vi "Init.vi"(8 "error in":errorcluster, 9 "Values":refnum<class "Value.lvclass">[](array[class]), 10 "Keys":refnum<class "Key Name.lvclass">[](array[class]), 11 "VAR in":refnum<class "VAR.lvclass">) -> (0 "error out":errorcluster, 3 "VAR out":refnum<class "VAR.lvclass">)   [LabVIEW 2020, in "Electronic Datasheet.lvlib" / "VAR.lvclass"]
uses:
  VAR.lvclass
  Keyname/Key Name.lvclass
  Value/Value.lvclass
  Object Type/Object Type Base.lvclass
  Electronic Datasheet.lvlib
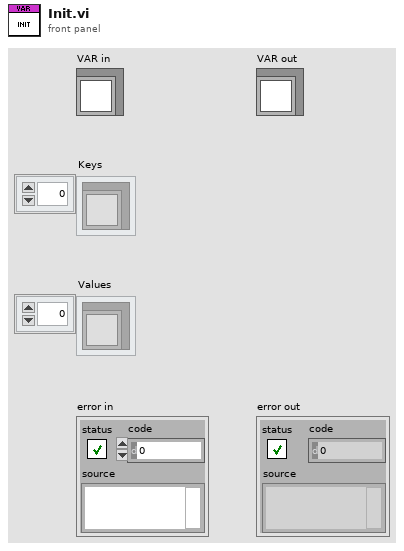
[diagram p1: front panel]
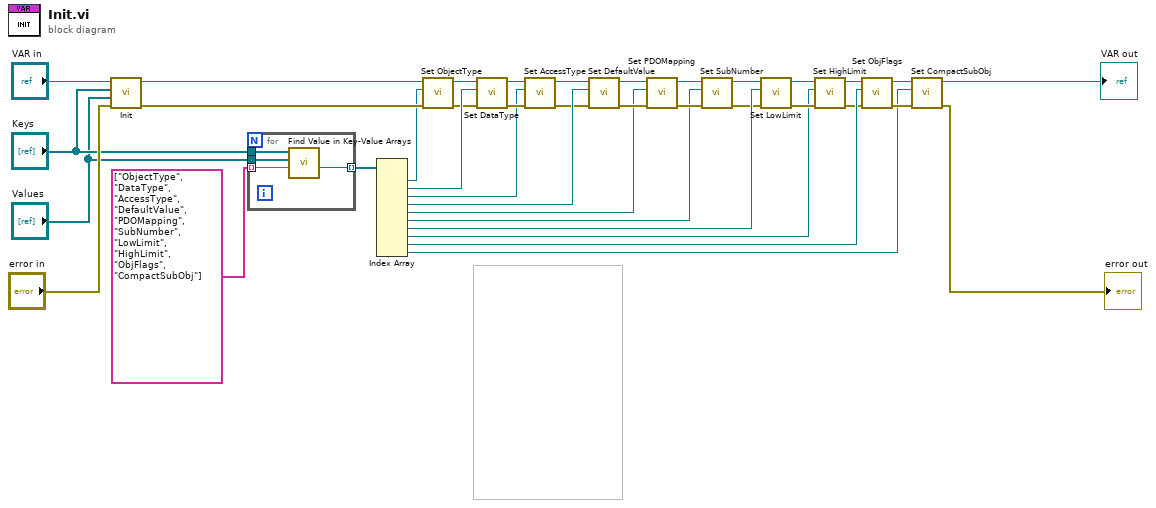
[diagram p0: block diagram]
diagram:
  n1 = call-parent "Init.vi"("error in"="error in", "Values"="Values", "Keys"="Keys", "Object Type in"="VAR in") -> ("error out"=w36:errorcluster, "Object Type out"=w3:refnum<class "VAR.lvclass">)  [unwired: 6 in]
  n2 = for {
    tunnel: "Keys" -> [w42]
    tunnel: "Values" -> [w41]
    tunnel: [w40] -> w32 mode=indexing
    tunnel: string[] ["ObjectType", "DataType", "AccessType", "DefaultValue", "PDOMapping", "SubNumber", "LowLimit", "HighLimit", "ObjFlags", "CompactSubObj"] -> [w39] mode=indexing
    n3 = call "Find Value in Key-Value Arrays.vi"("Key Name"=w39, "Values"=w41, "Keys"=w42) -> ("Value"=w40:refnum<class "Value.lvclass">)  [unwired: 5 in, 3 out]
  }
  n4 = Index Array(array=w32) -> (element #1=w1:refnum<class "Value.lvclass">, element #2=w31:refnum<class "Value.lvclass">, element #3=w28:refnum<class "Value.lvclass">, element #4=w27:refnum<class "Value.lvclass">, element #5=w22:refnum<class "Value.lvclass">, element #6=w19:refnum<class "Value.lvclass">, element #7=w17:refnum<class "Value.lvclass">, element #8=w14:refnum<class "Value.lvclass">, element #9=w12:refnum<class "Value.lvclass">, element #10=w8:refnum<class "Value.lvclass">)  [unwired: 10 in]
  n5 = call-dynamic "Set ObjectType.vi"("error in"=w36, "ObjectType"=w1, "Object Type in"=w3) -> ("error out"=w4:errorcluster, "Object Type out"=w2:refnum<class "VAR.lvclass">)  [unwired: 7 in]
  n6 = call-dynamic "Set DataType.vi"("error in"=w4, "Value"=w31, "Object Type in"=w2) -> ("error out"=w29:errorcluster, "Object Type out"=w33:refnum<class "VAR.lvclass">)  [unwired: 7 in]
  n7 = call-dynamic "Set AccessType.vi"("error in"=w29, "Value"=w28, "Object Type in"=w33) -> ("error out"=w26:errorcluster, "Object Type out"=w30:refnum<class "VAR.lvclass">)  [unwired: 7 in]
  n8 = call-dynamic "Set DefaultValue.vi"("error in"=w26, "Value"=w27, "Object Type in"=w30) -> ("error out"=w23:errorcluster, "Object Type out"=w25:refnum<class "VAR.lvclass">)  [unwired: 7 in]
  n9 = call-dynamic "Set PDOMapping.vi"("error in"=w23, "Value"=w22, "Object Type in"=w25) -> ("error out"=w20:errorcluster, "Object Type out"=w24:refnum<class "VAR.lvclass">)  [unwired: 7 in]
  n10 = call-dynamic "Set SubNumber.vi"("error in"=w20, "Value"=w19, "Object Type in"=w24) -> ("error out"=w5:errorcluster, "Object Type out"=w21:refnum<class "VAR.lvclass">)  [unwired: 7 in]
  n11 = call-dynamic "Set LowLimit.vi"("error in"=w5, "Value.lvclass"=w17, "Object Type in"=w21) -> ("error out"=w15:errorcluster, "Object Type out"=w18:refnum<class "VAR.lvclass">)  [unwired: 7 in]
  n12 = call-dynamic "Set HighLimit.vi"("error in"=w15, "Value"=w14, "Object Type in"=w18) -> ("error out"=w6:errorcluster, "Object Type out"=w16:refnum<class "VAR.lvclass">)  [unwired: 7 in]
  n13 = call-dynamic "Set ObjFlags.vi"("error in"=w6, "Value"=w12, "Object Type in"=w16) -> ("error out"=w9:errorcluster, "Object Type out"=w13:refnum<class "VAR.lvclass">)  [unwired: 7 in]
  n14 = call-dynamic "Set CompactSubObj.vi"("error in"=w9, "Value"=w8, "Object Type in"=w13) -> ("error out"=→"error out":errorcluster, "Object Type out"=→"VAR out":refnum<class "VAR.lvclass">)  [unwired: 7 in]
